vi "Keith 7001 Card Configure.vi"(1 "slot 2 # of poles (default:0)":u16(ring) items=["default", "1", "2", "4"], 2 "slot 2 card type (default:0)":u16(ring) items=["default", "none", "7052", "7053", "7054", "7056", "7057", "7058", "7059", "7061", "7062", "7063", "7064", "7065", "7066", "7067", "7152", "7153", "7154", "7156", "7158", "7164", "7166", "7168", "7169", "7402", "9990", "9991"], 3 "slot 2 delay (sec)":dbl min=0.0 max=99999.999 format="%.3f", 4 "card pairing":bool, 5 "slot 1 delay (sec)":dbl=-0.0 min=0.0 max=99999.999 format="%.3f", 6 "error in":T1, 7 "slot 1 # of poles (default:0)":u16(ring) items=["default", "1", "2", "4"], 8 "slot 1 card type (default:0)":u16(ring) items=["default", "none", "7052", "7053", "7054", "7056", "7057", "7058", "7059", "7061", "7062", "7063", "7064", "7065", "7066", "7067", "7152", "7153", "7154", "7156", "7158", "7164", "7166", "7168", "7169", "7402", "9990", "9991"], 9 "GPIB address":string="7") -> (0 "error out":T1)   [LabVIEW 2019]
doc: "This VI for the Keithley 7001 Switch System is used to configure the two card slots."
panel:
  # "on\noff"
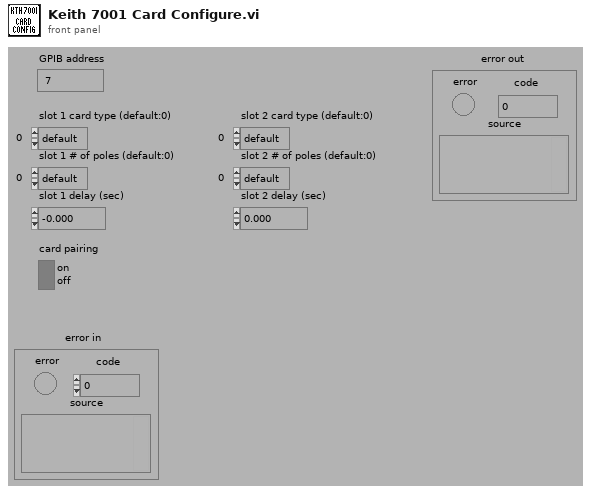
[diagram p1: front panel]
types:
  T1 = cluster{"error":bool, "code":i32, "source":string}
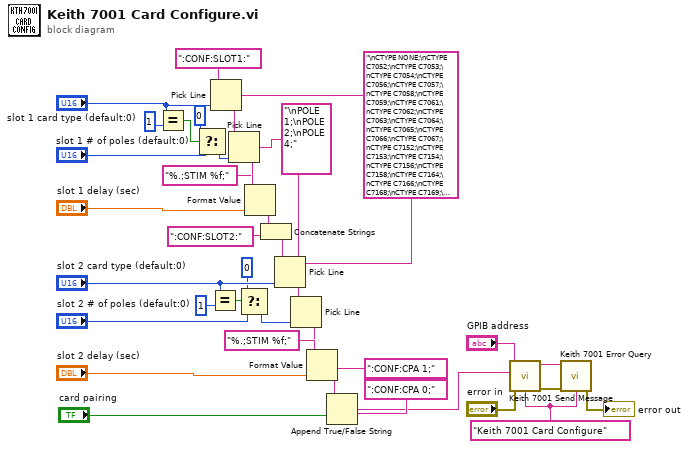
[diagram p0: block diagram]
diagram:
  w2 = "Keith 7001 Card Configure"
  w25 = "\nPOLE 1;\nPOLE 2;\nPOLE 4;"
  w26 = "\nCTYPE NONE;\nCTYPE C7052;\nCTYPE C7053;\nCTYPE C7054;\nCTYPE C7056;\nCTYPE C7057;\nCTYPE C7058;\nCTYPE C7059;\nCTYPE C7061;\nCTYPE C7062;\nCTYPE C7063;\nCTYPE C7064;\nCTYPE C7065;\nCTYPE C7066;\nCTYPE C7067;\nCTYPE C7152;\nCTYPE C7153;\nCTYPE C7154;\nCTYPE C7156;\nCTYPE C7158;\nCTYPE C7164;\nCTYPE C7166;\nCTYPE C7168;\nCTYPE C7169;\nCTYPE C7402;\nCTYPE C9990;\nCTYPE C9991;"
  n1 = Equal?(x="slot 1 card type (default:0)", y=1) -> (x = y?=w11:bool)
  n2 = Select(t=u16 0, s=w11, f="slot 1 # of poles (default:0)") -> (s? t:f=w16:u16)
  n3 = Equal?(x="slot 2 card type (default:0)", y=1) -> (x = y?=w9:bool)
  n4 = Pick Line(string ("")=":CONF:SLOT1:", multi-line string=w26, line index="slot 1 card type (default:0)") -> (output string=w36:string)
  n5 = Pick Line(string ("")=w36, multi-line string=w25, line index=w16) -> (output string=w35:string)
  n6 = Select(t=u16 0, s=w9, f="slot 2 # of poles (default:0)") -> (s? t:f=w14:u16)
  n7 = Format Value(string ("")=w35, format string="%.;STIM %f;", value (0)="slot 1 delay (sec)") -> (output string=w29:string)
  n8 = Concatenate Strings(w29, ":CONF:SLOT2:") -> (w27:string)
  n9 = Pick Line(string ("")=w27, multi-line string=w26, line index="slot 2 card type (default:0)") -> (output string=w30:string)
  n10 = Pick Line(string ("")=w30, multi-line string=w25, line index=w14) -> (output string=w31:string)
  n11 = Format Value(string ("")=w31, format string="%.;STIM %f;", value (0)="slot 2 delay (sec)") -> (output string=w23:string)
  n12 = Append True/False String(1:"card pairing", 2:":CONF:CPA 0;", 3:":CONF:CPA 1;", 4:w23) -> (0:w19:string)
  n13 = call "Keith 7001 Send Message.vi"("address string"="GPIB address", "write buffer"=w19, "source"=w2, "error in"="error in") -> ("address out"=w4:string, "error out"=w3:T1)  [unwired: 2 in, 2 out]
  n14 = call "Keith 7001 Error Query.vi"("GPIB address"=w4, "error in"=w3, "source"=w2) -> ("error out"=→"error out":T1)  [unwired: 2 out]
